vi "Win Msg Daemon.vi"(4 "error in (no error)":errorcluster, 5 "Messages (none)":u32[](array[numeric]), 6 "WinMsg Event":refnum<user-event>, 7 "VI Refnum":refnum<vi>) -> (0 "error out":errorcluster)   [LabVIEW 2011]
uses:
  Win Msg.ctl
panel:
  in  "WinMsg SYNC":T1
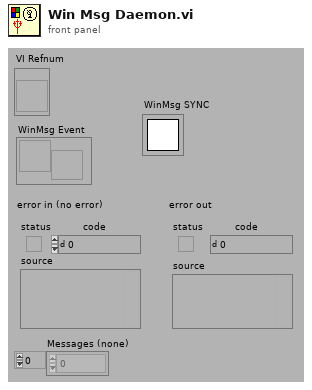
[diagram p1: front panel]
types:
  T1 = typedef "Rendezvous RefNum" = refnum<k1>
  T2 = typedef "Win Msg Q RefNum.ctl" = refnum<k1>
  T3 = typedef "Win Msg.ctl" = cluster{"hWnd":u32, "Msg":u32, "wParam":u32, "lParam":i32, "time":u32, "point":cluster{"X":i32, "Y":i32}}
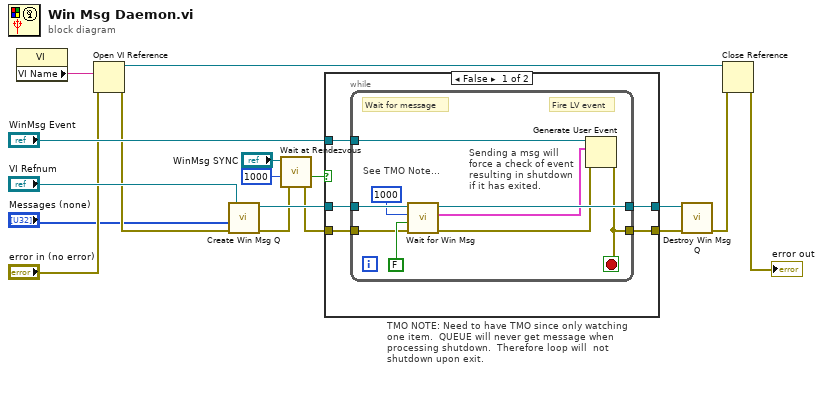
[diagram p0: block diagram]
diagram:
  # "TMO NOTE: Need to have TMO since only watching \none item.  QUEUE will never get message when processing shutdown.  Therefore loop will  not shutdown upon exit."
  n1 = property class="VI"() -> ("VI Name"=w12:string)  [unwired: 2 in, 2 out]
  n2 = Open VI Reference(vi path=w12, error in (no error)="error in (no error)") -> (vi reference=w11:refnum<vi>, error out=w7:errorcluster)  [unwired: 4 out]
  n3 = call "Create Win Msg Q.vi"("error in (no error)"=w7, "Messeges (none)"="Messages (none)", "VI Refnum"="VI Refnum") -> ("error out"=w6:errorcluster, "win msg queue"=w17:T2)  [unwired: 3 out]
  n4 = call <vilib>:"Wait at Rendezvous.vi"("error in (no error)"=w6, "ms timeout (-1)"=1000, "rendezvous"="WinMsg SYNC") -> ("error out"=w5:errorcluster, "timed out"=w2:bool)  [unwired: 3 out]
  n5 = case shown="False" w2 {
    tunnel: w17 -> [w22 w32]
    tunnel: [w21 w33] -> w16
    tunnel: [w20 w32] -> w15
    tunnel: "WinMsg Event" -> [w19 _]
    tunnel: w5 -> [w18 w33]
    frame False {
      n6 = while {
        tunnel: w18 -> [w29]
        tunnel: w22 -> [w30]
        tunnel: [w26] -> w21
        tunnel: [w28] -> w20
        tunnel: w19 -> [w25]
        stop <- w26 stop-if-true
        # "Sending a msg will \nforce a check of event\nresulting in shutdown\nif it has exited."
        # "See TMO Note..."
        # "Fire LV event"
        # "Wait for message"
        n7 = call "Wait for Win Msg.vi"("win msg queue"=w30, "ms timeout (-1)"=1000, "ignore previous (F)"=FALSE ("ignore previous (T)"), "error in (no error)"=w29) -> ("win msg queue out"=w28:T2, "Message"=w24:T3, "error out"=w27:errorcluster)  [unwired: 3 out]
        n8 = Generate User Event(user event=w25, event data cluster=w24, error in=w27) -> (error out=w26:errorcluster)  [unwired: 1 out]
      }
    }
    frame True {
    }
  }
  n9 = call "Destroy Win Msg Q.vi"("error in (no error)"=w16, "win msg queue"=w15) -> ("error out"=w10:errorcluster)  [unwired: 5 out]
  n10 = Close Reference(reference=w11, error in (no error)=w10) -> (error out=→"error out":errorcluster)
